vi "resize.vi"(1 "Array":u8[](array[numeric])) -> (0 "MIMIC_CMD":string)   [LabVIEW 2014]
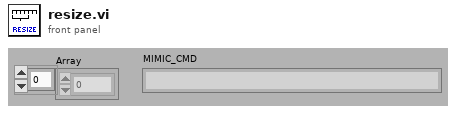
[diagram p1: front panel]
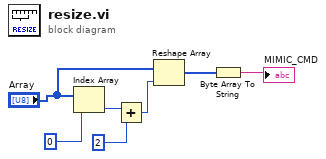
[diagram p0: block diagram]
diagram:
  n1 = Index Array(array="Array", index=0 ("Numeric")) -> (element=w2:u8)
  n2 = Add(x=w2, y=2) -> (x+y=w3:i32)
  n3 = Reshape Array("Array", w3) -> (w6:u8[])
  n4 = Byte Array To String(unsigned byte array=w6) -> (string=→"MIMIC_CMD":string)
